vi "Write Initialization VI Properties.vi"(8 "error in (no error)":errorcluster, 10 "Initialization VI Properties":T1={"Execution"=enum."silent", "Path"={"Path"=path "", "Path Type"=enum."Absolute"}, "Type"=enum."VI", "Position"=enum."centered"}, 11 "Initialization in":refnum<class "Initialization.lvclass">) -> (0 "error out":errorcluster, 3 "Initialization out":refnum<class "Initialization.lvclass">)   [LabVIEW 2015, in "Initialization.lvclass"]
uses:
  Initialization.lvclass
  Custom Device Type Defs/Initialization VI Properties.ctl
  XML Controls/Execution Types.ctl
  XML Controls/Path Cluster.ctl
  Initialization.lvclass/Initialization.ctl
  Configuration Tool.lvlib
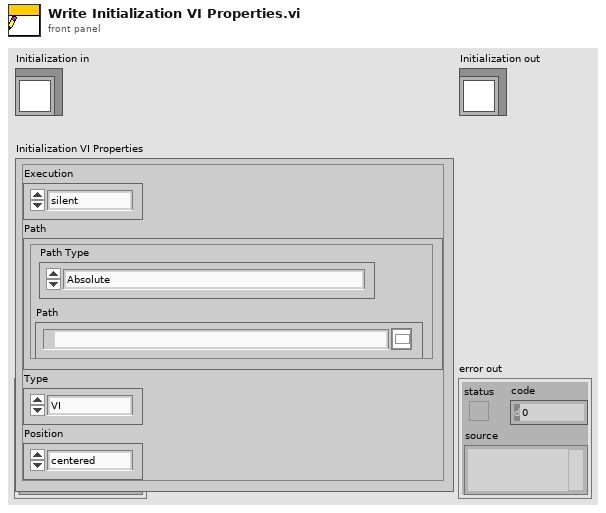
[diagram p1: front panel]
types:
  T1 = typedef "Initialization VI Properties.ctl" = cluster{"Execution":T2, "Path":T3, "Type":enum16{"Action", "VI"}, "Position":enum16{"centered", "mouse pointer"}}
  T2 = typedef "Configuration Tool.lvlib/Execution Types.ctl" = enum16{"silent", "modal", "floating", "default"}
  T3 = typedef "Configuration Tool.lvlib/Path Cluster.ctl" = cluster{"Path":path, "Path Type":enum16{"Absolute", "To Base", "To Common Doc Dir", "To Application Data Dir"}}
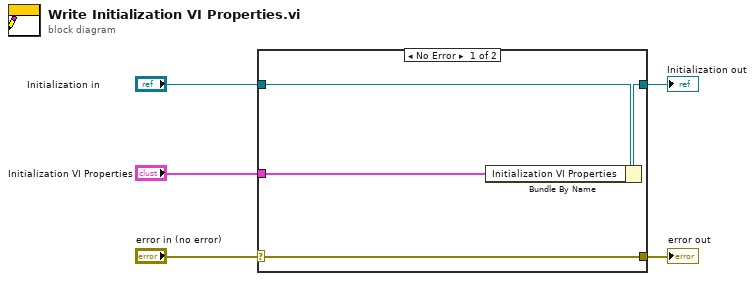
[diagram p0: block diagram]
diagram:
  n1 = case shown="No Error" "error in (no error)" {
    selector: "error in (no error)" -> [w9 w10]
    tunnel: [w9 w10] -> w4
    tunnel: [w7 w11] -> w2
    tunnel: "Initialization in" -> [w8 w11]
    tunnel: "Initialization VI Properties" -> [w6 _]
    frame No Error {
      n2 = Bundle By Name(cluster=w8, "Initialization VI Properties"=w6) -> (w7:refnum<class "Initialization.lvclass">)
    }
    frame Error {
    }
  }
  "error out" <- w4
  "Initialization out" <- w2
